vi "FRCts20_WebMethods_Competition_POST.vi"(7 "httpRequestID":u32) -> ()   [LabVIEW 2014]
doc: "<B>POST</B> a new competition resource\n\n<B>Required Data : </B>\n<Competition>\n <Name><B>string</B></Name>\n <Start_Date><B>YYYY-MM-DD</B></Start_Date>\n <Duration><B>uInt</B></Duration>\n</Competition>\n\nhttp://<server address>:<port>/FRCts/competition/\n\n{requires authentication}"
uses:
  FRCts20_WebMethods.lvlib
  Backend/source/VI Source/FRCts20_Backend_API/FRCts20_Backend_API.lvlib
  <vilib>/wsapi/NI_WebServices.lvlib
  FRCts20_WebMethods_ReadData_Events.vi
  Backend/source/VI Source/FRCts20_Backend_API/FRCts20_Backend_API_Event.vi
  Backend/source/VI Source/FRCts20_Backend_API/FRCts20_Backend_API_Event.ctl
  Backend/source/VI Source/FRCts20_Backend_API/FRCts20_Backend_API_SW.ctl
panel:
  in  "query":string
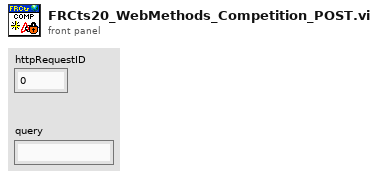
[diagram p1: front panel]
types:
  T1 = typedef "FRCts20_WebMethods.lvlib/FRCts20_WebMethods_ctl_singleEvent.ctl" = cluster{"Team":T2[], "Issue Count":i32, "Location":string, "Start Date ":timestamp}
  T2 = typedef "FRCts20_WebMethods.lvlib/FRCts20_WebMethods_ctl_teamIdentifier.ctl" = cluster{"Team Nickname":string, "Team Number ":u32, "UniqueId":u32}
  T3 = typedef "FRCts20_Backend_API.lvlib/FRCts20_Backend_API_Event.ctl" = cluster{"Event Index":u32, "Name":string, "Start Time":timestamp, "End Time":timestamp, "Teams":cluster{"Team Index":u32, "Team Number":u32, "Requests":cluster{"Request Number":u32, "Description":string}[], "Has Open Issue":bool}[], "SWType":T4, "APIReturn":string}
  T4 = typedef "FRCts20_Backend_API.lvlib/FRCts20_Backend_API_SW.ctl" = string
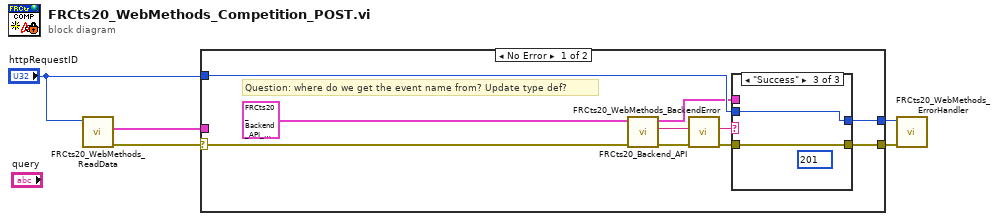
[diagram p0: block diagram]
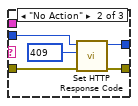
[diagram p3: hidden frame]
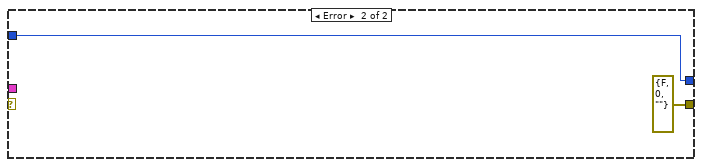
[diagram p4: hidden frame]
diagram:
  n1 = call-poly "FRCts20_WebMethods_ReadData.vi"("httpRequestID"="httpRequestID") -> ("error out"=w5:errorcluster, "Single Event out"=w4:T1)  [unwired: 8 in, 1 out]
  n2 = case shown="No Error" w5 {
    selector: w5 -> [w7 _]
    tunnel: w4 -> [_ _]
    tunnel: "httpRequestID" -> [w13 w26]
    tunnel: [w12 errorcluster {"status"=FALSE, "code"=0, "source"=""} ("error out")] -> w2
    tunnel: [w11 w26] -> w1
    frame No Error {
      # "Question: where do we get the event name from? Update type def?"
      n3 = call-poly "FRCts20_Backend_API.vi"("error in (no error)"=w7, "Event In"=T3 {"Event Index"=0, "Name"="", "Start Time"=timestamp(0 s since 1904-01-01), "End Time"=timestamp(0 s since 1904-01-01), "Teams"=[], "SWType"="", "APIReturn"=""}) -> ("error out"=w10:errorcluster, "Status"=w9:string, "Event Out"=w8:T3)  [unwired: 7 in]
      n4 = call "FRCts20_WebMethods_BackendError.vi"("error in (no error)"=w10, "Status"=w9) -> ("error out"=w14:errorcluster, "Status out"=w15:string)  [unwired: 8 in]
      n5 = case shown="\"Success\"" w15 {
        tunnel: w14 -> [w16 w19 w24]
        tunnel: w8 -> [_ _ _]
        tunnel: w13 -> [w17 w20 w23]
        tunnel: [w16 w22 w24] -> w12
        tunnel: [w17 w21 w23] -> w11
        frame "Backend Error", Default {
        }
        frame "No Action" {
          w18 = 409 items=["100"=100, "101"=101, "200"=200, "201"=201, "202"=202, "203"=203, "204"=204, "205"=205, "206"=206, "300"=300, "301"=301, "302"=302, "303"=303, "304"=304, "305"=305, "306"=306, "307"=307, "400"=400, "401"=401, "402"=402, "403"=403, "404"=404, "405"=405, "406"=406, "407"=407, "408"=408, "409"=409, "410"=410, "411"=411, "412"=412, "413"=413, "414"=414, "415"=415, "416"=416, "417"=417, "500"=500, "501"=501, "502"=502, "503"=503, "504"=504, "505"=505] ("response code (200)")
          n6 = call <vilib>:"Set HTTP Response Code.vi"("error in (no error)"=w19, "response code (200)"=w18, "httpRequestID"=w20) -> ("error out"=w22:errorcluster, "httpRequestID out"=w21:u32)  [unwired: 7 in]
        }
        frame "Success" {
          (unwired) 201 items=["100"=100, "101"=101, "200"=200, "201"=201, "202"=202, "203"=203, "204"=204, "205"=205, "206"=206, "300"=300, "301"=301, "302"=302, "303"=303, "304"=304, "305"=305, "306"=306, "307"=307, "400"=400, "401"=401, "402"=402, "403"=403, "404"=404, "405"=405, "406"=406, "407"=407, "408"=408, "409"=409, "410"=410, "411"=411, "412"=412, "413"=413, "414"=414, "415"=415, "416"=416, "417"=417, "500"=500, "501"=501, "502"=502, "503"=503, "504"=504, "505"=505] ("response code (200)")
        }
      }
    }
    frame Error {
    }
  }
  n7 = call "FRCts20_WebMethods_ErrorHandler.vi"("error in"=w2, "httpRequestID"=w1) -> ()  [unwired: 9 in, 1 out]
